vi "3_1_FiltroEMA.vi"() -> ()   [LabVIEW 2020]
uses:
  <vilib>/numeric/Random Number (Range) U64.vi
  <vilib>/numeric/sub_Random U32.vi
panel:
  out "Rojo=C°  Blanco=F° Verde=EMA":cluster{dbl, dbl, dbl}(graph)
  in  "Boolean 2":bool
  in  "Alpha":dbl=0.1
  out "Grados °C":cluster{dbl[], u64[]}(graph)
  out "Tabla de Grados":dbl[][](array[numeric])
  in  "Cantidad de \ngrados a crear":i32
  # "Centigrados"
  # "Farenheit"
  # "Filtro EMA"
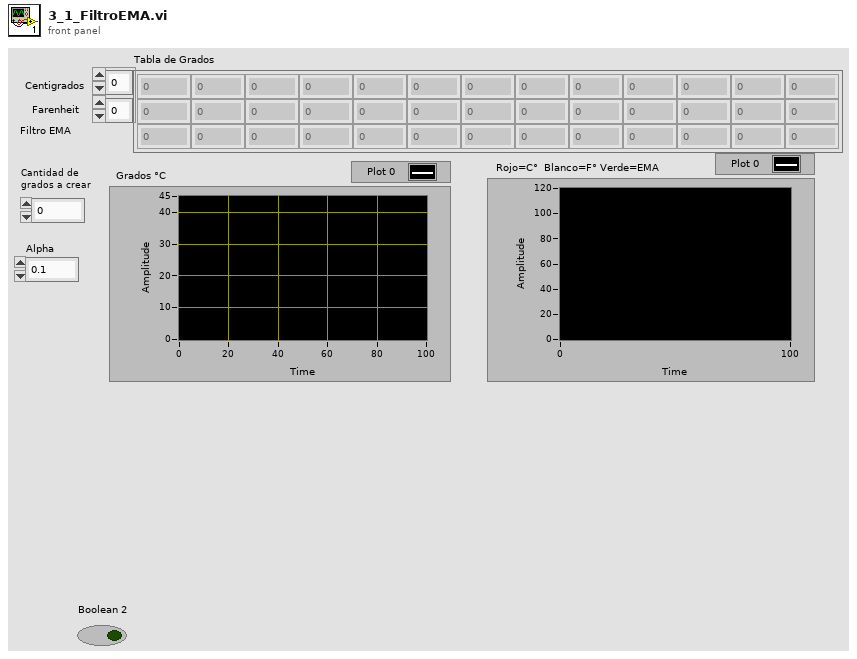
[diagram p1: front panel]
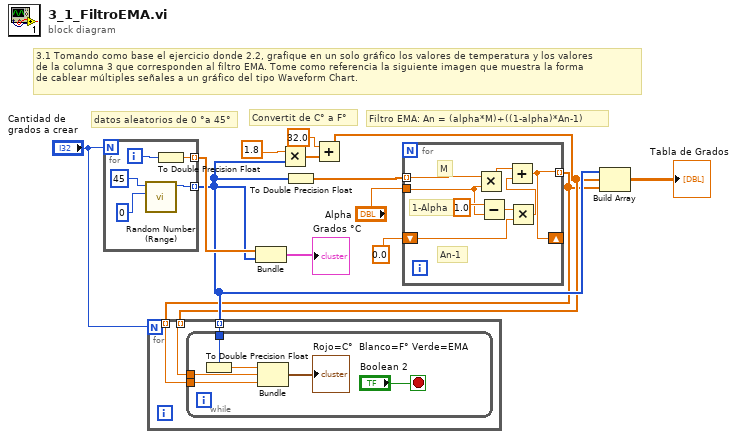
[diagram p0: block diagram]
diagram:
  # "Filtro EMA: An = (alpha*M)+((1-alpha)*An-1)"
  # "Convertit de C° a F°"
  # "datos aleatorios de 0 °a 45°"
  # "3.1 Tomando como base el ejercicio donde 2.2, grafique en un solo gráfico los valores de temperatura y los valores \nde la columna 3 que corresponden al filtro EMA. Tome como referencia la siguiente imagen que muestra la forma \nde cablear múltiples señales a un gráfico del tipo Waveform Chart."
  n1 = for {
    N: "Cantidad de \ngrados a crear" -> [_]
    tunnel: [w16] -> w4 mode=indexing
    tunnel: [w14] -> w10 mode=indexing
    i -> [w15]
    n2 = call-poly <vilib>:"Random Number (Range).vi"("lower bound (0)"=u64 0, "upper bound (100)"=u64 45) -> ("number"=w16:u64)  [unwired: 9 in]
    n3 = To Double Precision Float(number=w15) -> (double precision float=w14:dbl)
  }
  n4 = Bundle "Bundle"(w10, w4) -> (→"Grados °C":cluster{dbl[], u64[]})  [unwired: 1 in]
  n5 = Multiply(x=1.8, y=w4) -> (x*y=w12:dbl[])
  n6 = To Double Precision Float(number=w4) -> (double precision float=w8:dbl[])
  n7 = Add(x=32.0, y=w12) -> (x+y=w3:dbl[])
  n8 = for {
    tunnel: w8 -> [w25] mode=indexing
    shift-right: [w19] -> _
    shift-left: 0.0 -> [w23]
    tunnel: "Alpha" -> [w24]
    tunnel: [w19] -> w2 mode=indexing
    # "An-1"
    # "1-Alpha"
    # "M"
    n9 = Multiply(x=w25, y=w24) -> (x*y=w21:dbl)
    n10 = Subtract(x=1.0, y=w24) -> (x-y=w22:dbl)
    n11 = Multiply(x=w22, y=w23) -> (x*y=w20:dbl)
    n12 = Add(x=w21, y=w20) -> (x+y=w19:dbl)
  }
  n13 = for {
    N: "Cantidad de \ngrados a crear" -> [_]
    tunnel: w4 -> [w29] mode=indexing
    tunnel: w3 -> [w28] mode=indexing
    tunnel: w2 -> [w27] mode=indexing
    n14 = while {
      tunnel: w29 -> [w33]
      tunnel: w28 -> [w35]
      tunnel: w27 -> [w34]
      stop <- "Boolean 2" stop-if-true
      n15 = To Double Precision Float(number=w33) -> (double precision float=w30:dbl)
      n16 = Bundle "Bundle"(w30, w35, w34) -> (→"Rojo=C°  Blanco=F° Verde=EMA":cluster{dbl, dbl, dbl})  [unwired: 1 in]
    }
  }
  n17 = Build Array "Build Array"(w4, w3, w2) -> (→"Tabla de Grados":dbl[][])
